vi "pythonArrayTest.vi"() -> ()   [LabVIEW 2017]
panel:
  in  "stop":bool
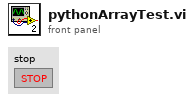
[diagram p1: front panel]
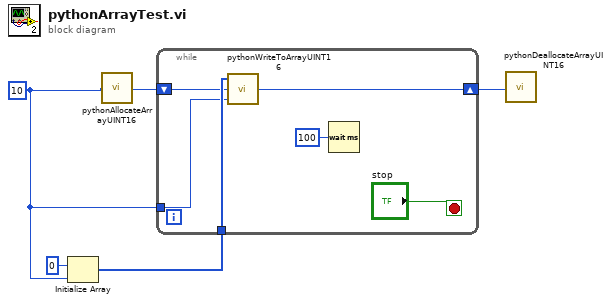
[diagram p0: block diagram]
diagram:
  w2 = 10 ("size")
  n1 = Initialize Array(u16 0 ("element"), w2) -> (w4:u16[])
  n2 = call "pythonAllocateArrayUINT16.vi"("size"=w2) -> ("pointer"=w3:i64)
  n3 = while {
    tunnel: w4 -> [w11]
    tunnel: w2 -> [w9]
    shift-right: [w8] -> w1
    shift-left: w3 -> [w10]
    stop <- "stop" stop-if-true
    n4 = call "pythonWriteToArrayUINT16.vi"("size"=w9, "dst"=w10, "src"=w11) -> ("dst out"=w8:i64)
    n5 = Wait (ms)(milliseconds to wait=u32 100) -> ()  [unwired: 1 out]
  }
  n6 = call "pythonDeallocateArrayUINT16.vi"("ptr"=w1) -> ()  [unwired: 1 in]
